vi "List errors.vi"(3 "XRef":refnum<vi>, 4 "State In":T1, 5 "Generate Strings?":bool) -> (0 "Errors Present?":bool, 1 "Errors":string[](array[string]), 2 "Details":string[](array[string]))   [LabVIEW 2012]
uses:
  State.ctl
  FilterArray.xnode
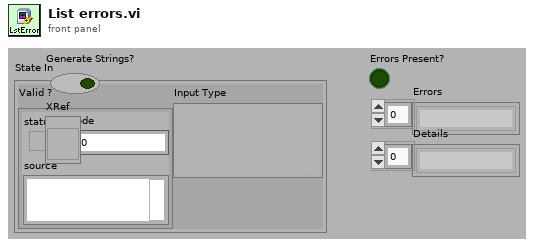
[diagram p1: front panel]
types:
  T1 = typedef "FilterArray.xnode/State.ctl" = cluster{"Valid ?":errorcluster, "Input Type":variant}
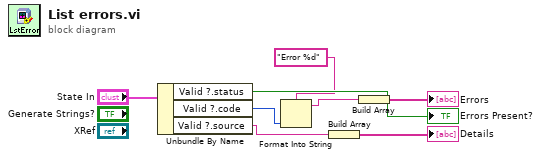
[diagram p0: block diagram]
diagram:
  n1 = Unbundle By Name("State In") -> ("Valid ?.status"=→"Errors Present?":bool, "Valid ?.code"=w5:i32, "Valid ?.source"=w2:string)
  n2 = Format Into String(format string="Error %d", w5) -> (resulting string=w4:string)  [unwired: 2 in, 1 out]
  n3 = Build Array(w2) -> (→"Details":string[])
  n4 = Build Array(w4) -> (→"Errors":string[])
